vi "Get image dimensions from Tiff file.vi"(8 "error in":errorcluster, 11 "path to TIFF file":path=path "C:/Users/dmilkie/Desktop/stack.tif") -> (0 "error out":errorcluster, 1 "Y Size":u32, 2 "X Size":u32, 3 "path to TIFF file dup":path=path "C:/Users/dmilkie/Desktop/stack.tif")   [LabVIEW 2013, in "Tiff reader.lvlib"]
uses:
  Tiff reader.lvlib
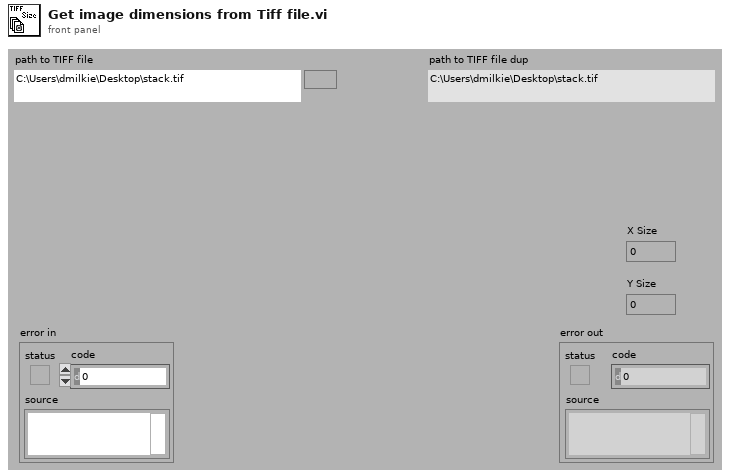
[diagram p1: front panel]
types:
  T1 = enum16{"open", "replace", "create", "open or create", "replace or create", "replace or create with confirmation"}
  T2 = typedef "Tiff reader.lvlib/IFD Entry.ctl" = cluster{"Tag":u16, "Type":T3, "Count":u32, "Val/Offs":u32, "Is Pointer?":bool, "Byte stream index":i32}
  T3 = typedef "Tiff reader.lvlib/FieldTypes.ctl" = enum16{"NULL", "U8", "ASCII7", "U16", "U32", "RATIONAL", "SByte(I8)", "Undef(8Bit)", "I16", "I32", "SRat(4B:4B)", "SGL(4Byte)", "DBL(8Byte)"}
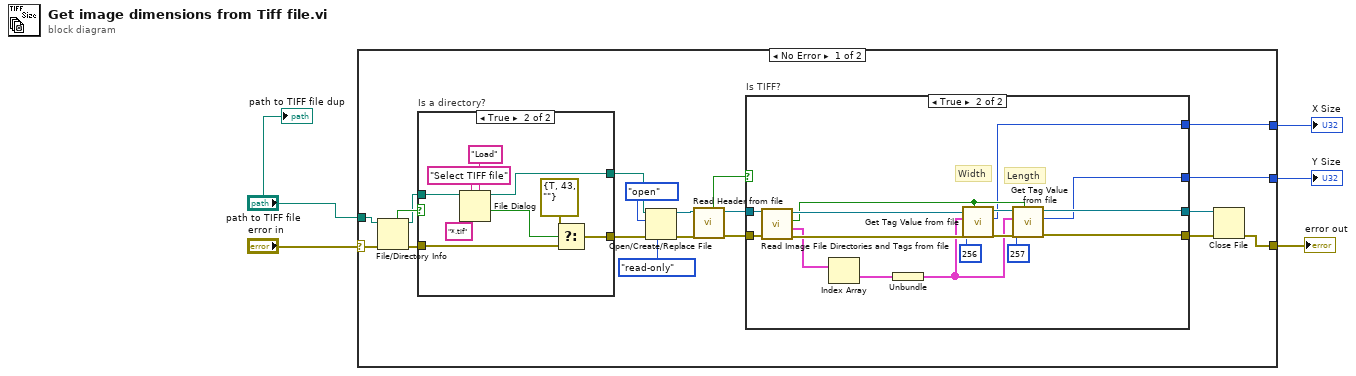
[diagram p0: block diagram]
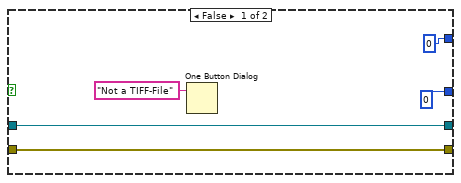
[diagram p2: hidden frame]
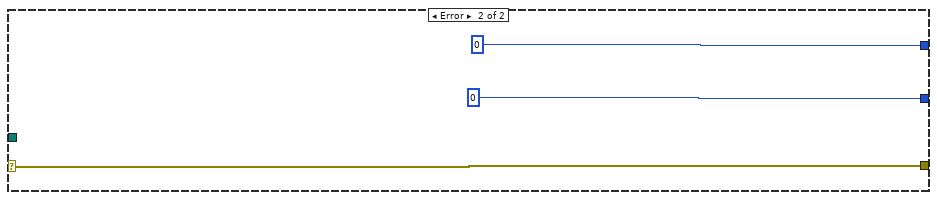
[diagram p4: hidden frame]
diagram:
  n1 = case shown="No Error" "error in" {
    selector: "error in" -> [w15 w59]
    tunnel: "path to TIFF file" -> [w23 _]
    tunnel: [w9 w59] -> w4
    tunnel: [w7 u32 0 ("Single Value")] -> w3
    tunnel: [w6 u32 0 ("Single Value")] -> w2
    frame No Error {
      n2 = File/Directory Info(path=w23, error in=w15) -> (path out=w14:path, directory=w24:bool, error out=w22:errorcluster)  [unwired: 4 out]
      n3 = case "Is a directory?" shown="True" w24 {
        tunnel: w22 -> [w47 w53]
        tunnel: w14 -> [w46 w52]
        tunnel: [w47 w48] -> w18
        tunnel: [w46 w49] -> w17
        frame False {
        }
        frame True {
          n4 = File Dialog(5:"Load" ("button label"), 6:"*.tif" ("pattern"), 7:"Select TIFF file" ("prompt"), 11:w52) -> (1:w54:bool, 3:w49:path)  [unwired: 1 in, 4 out]
          n5 = Select(t=errorcluster {"status"=TRUE, "code"=43, "source"=""} ("error in (no error)"), s=w54, f=w53) -> (s? t:f=w48:errorcluster)
        }
      }
      n6 = Open/Create/Replace File(file path (use dialog)=w17, error in=w18, operation (0:open)=T1."open", access (0:read/write)=enum16{"read/write", "read-only", "write-only"}."read-only") -> (refnum out=w16:refnum<file>, error out=w19:errorcluster)  [unwired: 3 out]
      n7 = call "Read Header from file.vi"("error in"=w19, "File"=w16) -> ("error out"=w12:errorcluster, "File"=w13:refnum<file>, "isTIFF"=w11:bool)  [unwired: 5 out]
      n8 = case "Is TIFF?" shown="True" w11 {
        tunnel: [w28 w34] -> w10
        tunnel: w13 -> [w27 w45]
        tunnel: w12 -> [w28 w44]
        tunnel: [w27 w41] -> w8
        tunnel: [u32 0 ("Single Value") w31] -> w7
        tunnel: [u32 0 ("Single Value") w30] -> w6
        frame False {
          n9 = One Button Dialog(message="Not a TIFF-File") -> ()  [unwired: 2 out]
        }
        frame True {
          # "Length"
          # "Width"
          n10 = call "Read Image File Directories and Tags from file.vi"("error in"=w44, "File"=w45) -> ("error out"=w42:errorcluster, "Tags for each IFD"=w40:cluster{"Tags":T2[]}[], "Litt/BigEnd"=w33:bool, "File"=w43:refnum<file>)  [unwired: 2 out]
          n11 = Index Array(array=w40) -> (element=w39:cluster{"Tags":T2[]})  [unwired: 1 in]
          n12 = Unbundle(w39) -> ("Tags"=w32:T2[])
          n13 = call "Get Tag Value from file.vi"("Litt/BigEnd"=w33, "error in"=w42, "Tag Code"=u16 256, "DirEntries"=w32, "File"=w43) -> ("error out"=w36:errorcluster, "Single Value"=w31:u32, "File"=w38:refnum<file>)  [unwired: 4 out]
          n14 = call "Get Tag Value from file.vi"("Litt/BigEnd"=w33, "error in"=w36, "Tag Code"=u16 257, "DirEntries"=w32, "File"=w38) -> ("error out"=w34:errorcluster, "Single Value"=w30:u32, "File"=w41:refnum<file>)  [unwired: 4 out]
        }
      }
      n15 = Close File(refnum=w8, error in=w10) -> (error out=w9:errorcluster)  [unwired: 1 out]
    }
    frame Error {
    }
  }
  "error out" <- w4
  "X Size" <- w3
  "Y Size" <- w2
  "path to TIFF file dup" <- "path to TIFF file"
